vi "Graves Count.vi"(8 "Error In":errorcluster, 11 "Test Target In":refnum<vi>) -> (0 "Error Out":errorcluster, 2 "Graves Count":i32, 3 "Test Target Out":refnum<vi>)   [LabVIEW 2018, in "Tests.lvlib" / "Toolkit.lvlib" / "Integration.lvlib"]
uses:
  Integration.lvlib
  src/Toolkit/Toolkit.lvlib
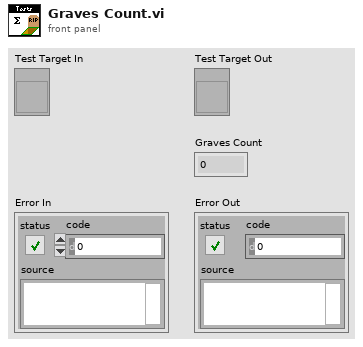
[diagram p1: front panel]
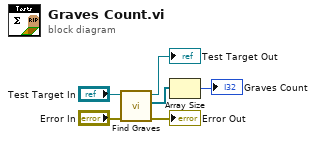
[diagram p0: block diagram]
diagram:
  n1 = call "Find Graves.vi"("Error In"="Error In", "VI In"="Test Target In") -> ("Error Out"=→"Error Out":errorcluster, "Graves"=w4:refnum<vi>[], "VI Out"=→"Test Target Out":refnum<vi>)  [unwired: 7 in]
  n2 = Array Size(array=w4) -> (size(s)=→"Graves Count":i32)
